vi "5-3 ordine crescente vettori.vi"(0 "Vettore iniziale":dbl[](array[numeric])=[1.0, -2.0, 6.0, -5.0, -1.0, 7.0] format="%.2f") -> (1 "array ordinato":dbl[](array[numeric]) format="%.2f", 2 "vettore riordinato":dbl[](array[numeric]) format="%.2f")   [LabVIEW 2012]
panel:
  # "Ordinare in modo crescente il vettore iniziale"
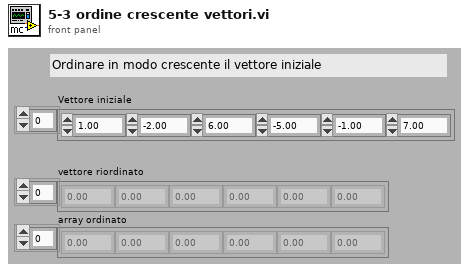
[diagram p1: front panel]
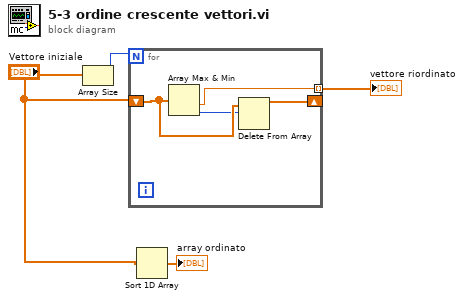
[diagram p0: block diagram]
diagram:
  n1 = Array Size(array="Vettore iniziale") -> (size(s)=w4:i32)
  n2 = for {
    N: w4 -> [_]
    shift-right: [w7] -> _
    shift-left: "Vettore iniziale" -> [w8]
    tunnel: [w5] -> w1 mode=indexing
    n3 = Array Max & Min(array=w8) -> (min value=w5:dbl, min index (indices)=w6:i32)  [unwired: 2 out]
    n4 = Delete From Array(array=w8, index=w6) -> (array with subset deleted=w7:dbl[])  [unwired: 1 in, 1 out]
  }
  "vettore riordinato" <- w1
  n5 = Sort 1D Array(array="Vettore iniziale") -> (sorted array=→"array ordinato":dbl[])
